vi "sendInfoLoopToLoop.vi"(11 "scan info":T1) -> (0 "num empty spaces for commands":u32, 1 "num successful commands looped":u32, 2 "codeOutOfRange":bool, 3 "numLoopToLoopErrors":u32)   [LabVIEW 2010]
uses:
  scan_command.ctl
  scan message.ctl
  <vilib>/rvi/DataTransferAndStorage/Container/XNode/niFpgaContainer.xnode
  <vilib>/rvi/FIFO/Fifo_Resource/nirvififoEmulationSetSize.vi
  <vilib>/rvi/DataTransferAndStorage/Container/Common/niFpgaContainerGetUniqueNameForEmu.vi
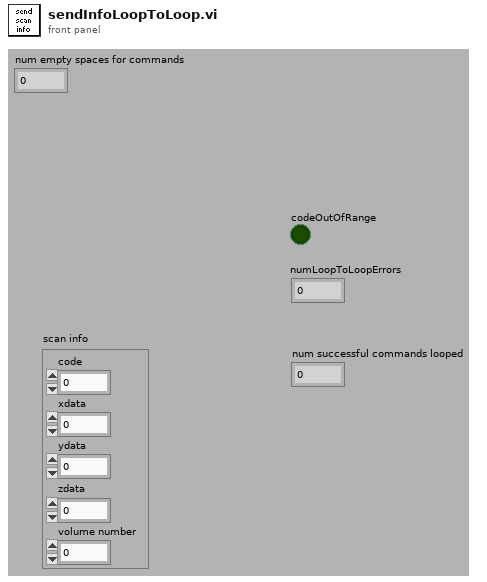
[diagram p1: front panel]
types:
  T1 = typedef "scan_command.ctl" = cluster{"code":i32, "xdata":i32, "ydata":i32, "zdata":i32, "volume number":i32}
  T2 = typedef "scan message.ctl" = enum16{"NONE", "VOLUME START", "LINE START", "COM"}
  T3 = cluster{"code":i32, "xdata":i32, "ydata":i32, "zdata":i32, "volume number":i32}
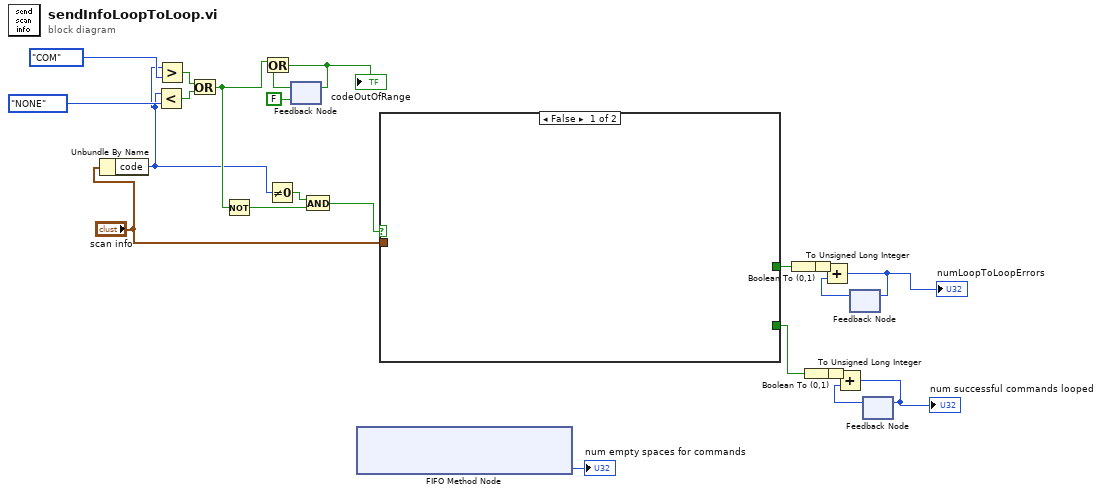
[diagram p0: block diagram]
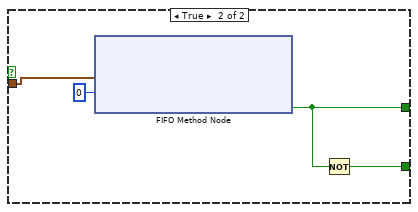
[diagram p2: hidden frame]
diagram:
  n1 = Unbundle By Name("scan info") -> ("code"=w10:i32)
  n2 = Less?(x=w10, y=scan_message."NONE" ("Enum")) -> (x < y?=w20:bool)
  n3 = Greater?(x=w10, y=scan_message."COM" ("Enum")) -> (0:w21:bool)
  n4 = Or(x=w21, y=w20) -> (x .or. y?=w11:bool)
  n5 = Not(x=w11) -> (.not. x?=w1:bool)
  n6 = Not Equal To 0?(x=w10) -> (x != 0?=w8:bool)
  n7 = feedback #1(FALSE) -> (w17:bool)
  n8 = Or(x=w11, y=w17) -> (x .or. y?=w19:bool)
  "codeOutOfRange" <- w19
  n9 = feedback-in #1(w19) -> ()
  n10 = And(x=w8, y=w1) -> (x .and. y?=w9:bool)
  n11 = xnode ("FIFO Method Node")() -> ("Number of Elements to Write"=→"num empty spaces for commands":u32)  [unwired: 1 in, 1 out]
  n12 = case shown="False" w9 {
    tunnel: "scan info" -> [_ w27]
    tunnel: [_ w26] -> w24
    tunnel: [_ w25] -> w3
    frame False {
    }
    frame True {
      n13 = xnode ("FIFO Method Node")("Element"=w27, "Timeout"=0) -> ("Timed Out?"=w26:bool)  [unwired: 1 in, 1 out]
      n14 = Not(x=w26) -> (.not. x?=w25:bool)
    }
  }
  n15 = Boolean To (0,1)(Boolean=w24) -> (0, 1=w16:i16)
  n16 = Boolean To (0,1)(Boolean=w3) -> (0, 1=w5:i16)
  n17 = To Unsigned Long Integer(number=w16) -> (unsigned 32bit integer=w15:u32)
  n18 = To Unsigned Long Integer(number=w5) -> (unsigned 32bit integer=w4:u32)
  n19 = feedback #2() -> (w22:u32)  [unwired: 1 in]
  n20 = Add(x=w15, y=w22) -> (x+y=w23:u32)
  "numLoopToLoopErrors" <- w23
  n21 = feedback-in #2(w23) -> ()
  n22 = feedback #3() -> (w6:u32)  [unwired: 1 in]
  n23 = Add(x=w4, y=w6) -> (x+y=w7:u32)
  "num successful commands looped" <- w7
  n24 = feedback-in #3(w7) -> ()
